vi "TestVIServer.vi"   [LabVIEW 2015]
types:
  T1 = enum32{"Invalid", "Standard", "Closed", "Hidden", "Minimized", "Maximized"}
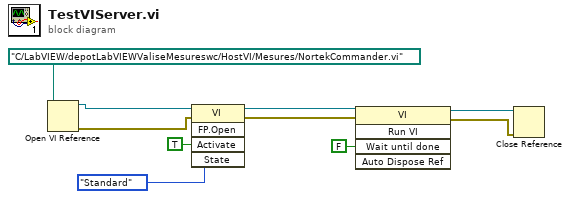
[diagram p0: block diagram]
diagram:
  n1 = Open VI Reference(vi path=path "C:/LabVIEW/depotLabVIEWValiseMesureswc/HostVI/Mesures/NortekCommander.vi") -> (vi reference=w9:refnum<vi>, error out=w8:errorcluster)  [unwired: 5 in]
  n2 = invoke class="VI" method="FP.Open"(reference=w9, error in=w8, "Activate"=TRUE ("Activate?"), "State"=T1."Standard") -> (reference out=w6:refnum<vi>, error out=w7:errorcluster)  [unwired: 1 in, 3 out]
  n3 = invoke class="VI" method="Run VI"(reference=w6, error in=w7, "Wait until done"=FALSE ("Wait Until Done")) -> (reference out=w5:refnum<vi>, error out=w4:errorcluster)  [unwired: 2 in, 3 out]
  n4 = Close Reference(reference=w5, error in (no error)=w4) -> ()  [unwired: 1 out]
